vi "Set FP Panel Bounds.vi"(8 "error in (no error)":errorcluster, 10 "FP panel bounds":T1, 11 "VI Panel Layout in":refnum<class "VI Panel Layout.lvclass">) -> (0 "error out":errorcluster, 3 "VI Panel Layout out":refnum<class "VI Panel Layout.lvclass">)   [LabVIEW 2010, in "NI_SE_Front Panel Layout.lvlib" / "VI Panel Layout.lvclass"]
uses:
  VI Panel Layout.lvclass
  <vilib>/Utility/miscctls.llb/LVRectTypeDef.ctl
  VI Panel Layout.lvclass/VI Panel Layout.ctl
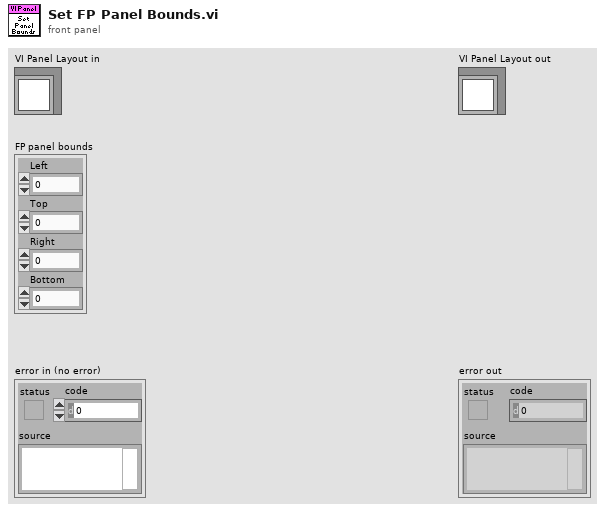
[diagram p1: front panel]
types:
  T1 = typedef "LVRectTypeDef.ctl" = cluster{"Left":i16, "Top":i16, "Right":i16, "Bottom":i16}
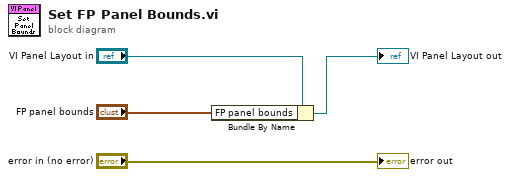
[diagram p0: block diagram]
diagram:
  n1 = Bundle By Name(cluster="VI Panel Layout in", "FP panel bounds"="FP panel bounds") -> (→"VI Panel Layout out":refnum<class "VI Panel Layout.lvclass">)
  "error out" <- "error in (no error)"
